vi "Nonlinear Calibration Test v2.vi"() -> ()   [LabVIEW 2009]
doc: "This example illustrates the use of a calibration grid to calibrate and correct an image for nonlinear distortion and accurate shape measurements.\n\nThis example loads the image of a calibration grid used to calibrate the system, learns the grid, then loads an image of parts acquired using the same setup. The example then corrects the image in two ways. The first method corrects the entire image and then measures the area of the coins. The second method corrects only the area of the coins and displays the difference in processing time."
uses:
  <vilib>/vision/NI_Vision_Development_Module.lvlib
panel:
  in  "Grid Descriptor":T1={"X Step"=1.0, "Y Step"=1.0, "Unit"=enum."Undefined", "Threshold Range"={"Lower value"=30.0, "Upper value"=96.0}} {"Threshold Range"."Upper value" format="%.2f"; "Threshold Range"."Lower value" format="%.2f"; "Y Step" format="%.2f"; "X Step" format="%.2f"}
  in  "Calibration Learn Setup":T3={"Distortion"=0, "Corrected Image Scaling"=0, "Corrected Image Learn ROI"=2, "Learn Error Map?"=FALSE, "Learn Correction Table?"=FALSE} {"Corrected Image Learn ROI" items=["Full Image ", "Calibration ROI", "ROI", "Calibration AND ROI", "Calibration OR ROI"]; "Corrected Image Scaling" items=["Scale to Preserve Area", "Scale to Fit"]; "Distortion" items=["Perspective", "Nonlinear"]}
  out "Bottom Image":T4(plugin-control) caption="Coins Image"
  out "Top Image":T4(plugin-control) caption="Calibration Template"
  # "1. Loads the image of a calibration grid that is used to calibrate the system."
  # "2. Learn the calibration grid. Note that this process is computation intensive and needs a fair amount of time to complete."
  # "3. Load Image of Parts acquired using the same setup."
  # "4. Correct the image and measure areas of the objects in the image."
  # "This step takes measurements in two ways.  The first calculation corrects \nthe entire image, and then takes the measurements.  The second calculation only corrects the coins, and then takes the measurements."
  # "time (ms) to correct entire image, threshold and calculate measurements"
  # "time (ms) to threshold, correct just coins, and then take measurements"
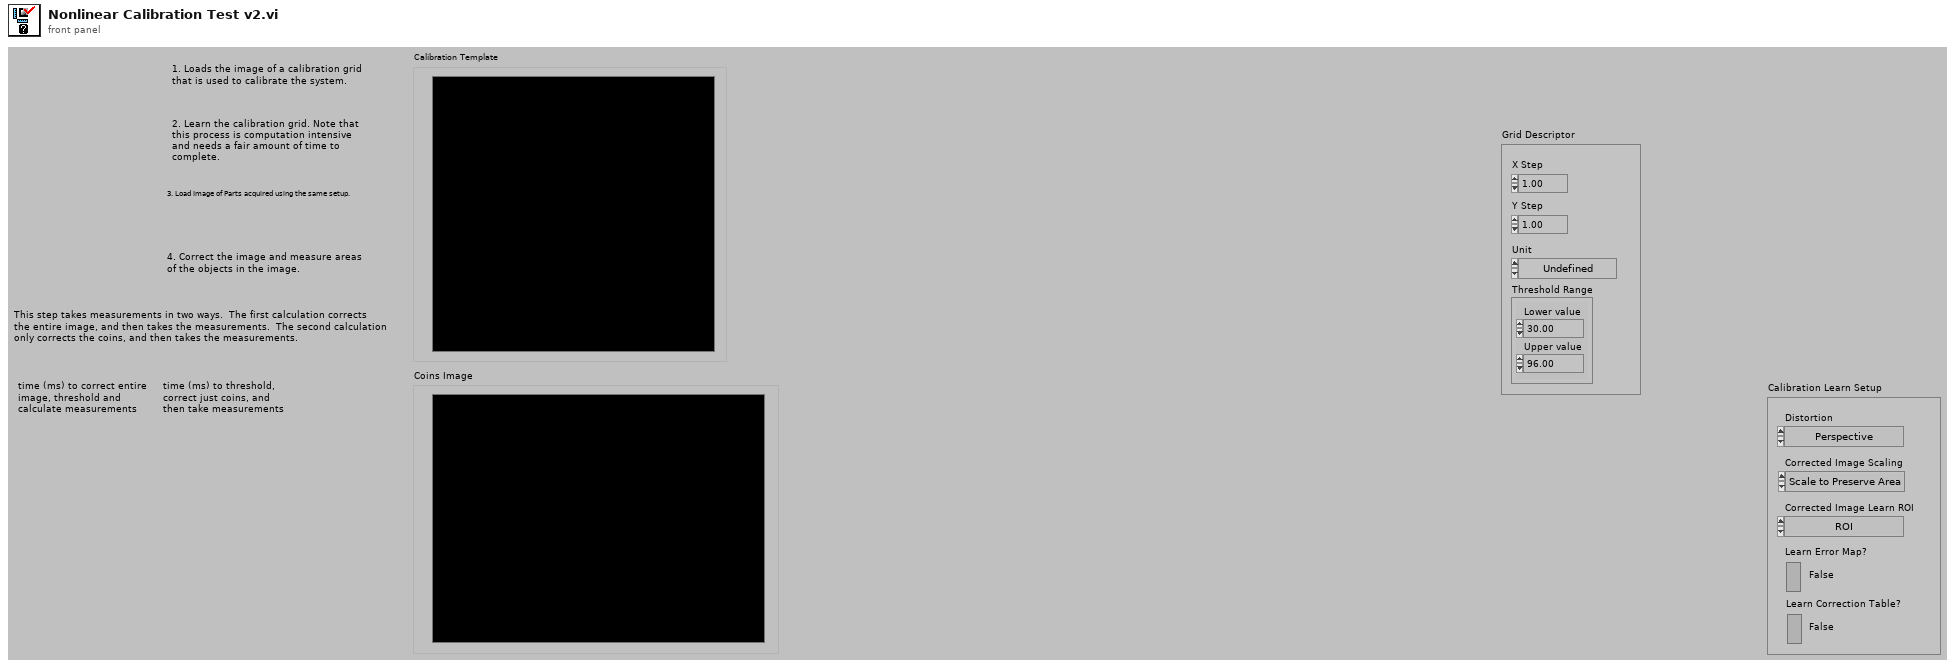
[diagram p1: front panel]
types:
  T1 = typedef "Grid Descriptor" = cluster{"X Step":sgl, "Y Step":sgl, "Unit":T2, "Threshold Range":cluster{"Lower value":sgl, "Upper value":sgl}}
  T2 = typedef "Image Unit" = enum32{"Undefined", "Angström", "Micrometer", "Millimeter", "Centimeter", "Meter", "Kilometer", "Microinch", "Inch", "Feet", "Nautical miles", "Standard miles", "Steps"}
  T3 = cluster{"Distortion":u32, "Corrected Image Scaling":u32, "Corrected Image Learn ROI":u32, "Learn Error Map?":bool, "Learn Correction Table?":bool}
  T4 = typedef "IMAQ Image.ctl" = refnum<image>
  T5 = cluster{"X Step":sgl, "Y Step":sgl, "Unit":u32, "Threshold Range":cluster{"Lower value":sgl, "Upper value":sgl}}
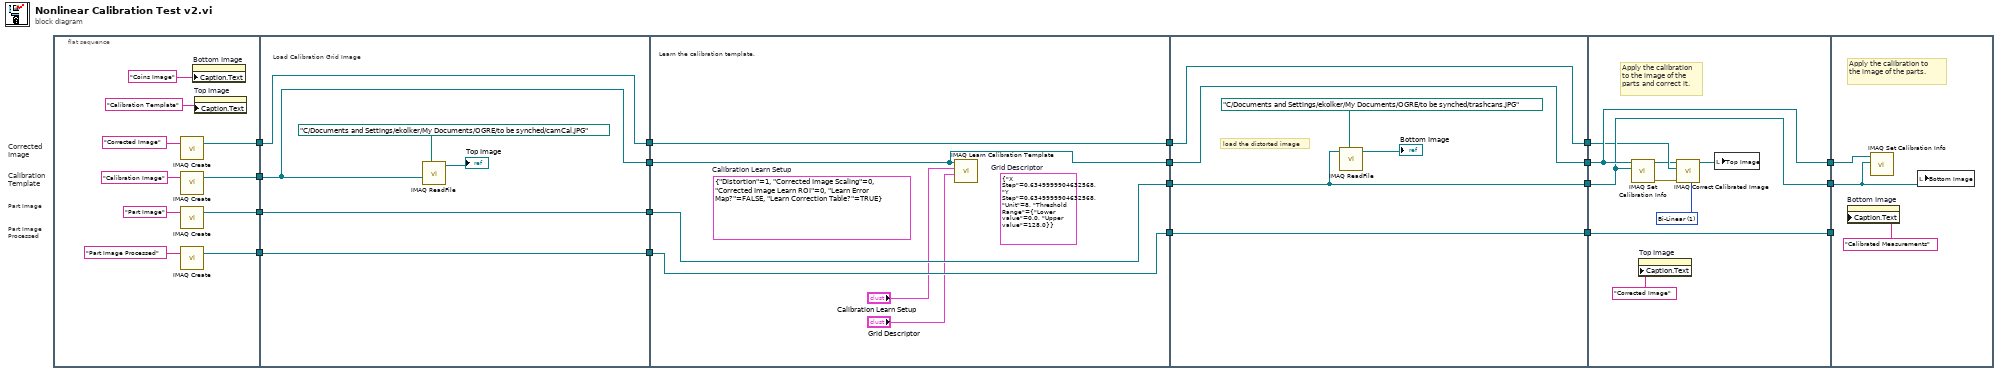
[diagram p0: block diagram]
diagram:
  # "Corrected\nImage"
  # "Part Image Processed"
  # "Calibration Template"
  # "Part Image"
  n1 = flat-sequence {
    tunnel: [w28] -> w19
    tunnel: [w26] -> w18
    tunnel: [w24] -> w17
    tunnel: [w22] -> w16
    tunnel: w19 -> [w35]
    tunnel: [w35] -> w12
    tunnel: w18 -> [w32]
    tunnel: [w32] -> w11
    tunnel: w17 -> [w34]
    tunnel: [w34] -> w10
    tunnel: w16 -> [w33]
    tunnel: [w33] -> w9
    tunnel: w12 -> [w40]
    tunnel: [w40] -> w8
    tunnel: w11 -> [w41]
    tunnel: [w41] -> w7
    tunnel: w10 -> [w39]
    tunnel: [w39] -> w6
    tunnel: w9 -> [w38]
    tunnel: [w38] -> w5
    tunnel: w8 -> [w47]
    tunnel: [w47] -> w4
    tunnel: w7 -> [w45]
    tunnel: [w45] -> w3
    tunnel: w6 -> [w44]
    tunnel: [w44] -> w2
    tunnel: w5 -> [w43]
    tunnel: [w43] -> w1
    tunnel: w4 -> [w55]
    tunnel: [w55] -> w15
    tunnel: w3 -> [w56]
    tunnel: [w56] -> w14
    tunnel: w2 -> [w54]
    tunnel: [w54] -> w13
    tunnel: w1 -> [w53]
    tunnel: w15 -> [w57]
    tunnel: w14 -> [w59]
    tunnel: w13 -> [_]
    frame #0 {
      # "Create the required images"
      n2 = call "IMAQ Create"("Image Name"="Corrected Image") -> ("New Image"=w22:T4)  [unwired: 3 in, 2 out]
      n3 = call "IMAQ Create"("Image Name"="Calibration Image") -> ("New Image"=w26:T4)  [unwired: 3 in, 2 out]
      n4 = call "IMAQ Create"("Image Name"="Part Image") -> ("New Image"=w28:T4)  [unwired: 3 in, 2 out]
      n5 = call "IMAQ Create"("Image Name"="Part Image Processed") -> ("New Image"=w24:T4)  [unwired: 3 in, 2 out]
      n6 = property on="Bottom Image" class="ImageControl"("Caption.Text"="Coins Image" ("Title")) -> ()  [unwired: 2 in, 2 out]
      n7 = property on="Top Image" class="ImageControl"("Caption.Text"="Calibration Template" ("Title")) -> ()  [unwired: 2 in, 2 out]
    }
    frame #1 {
      # "Load Calibration Grid Image"
      n8 = call "IMAQ ReadFile"("File Path"=path "C:/Documents and Settings/ekolker/My Documents/OGRE/to be synched/camCal.JPG", "Image"=w32) -> ("Image Out"=→"Top Image":T4)  [unwired: 3 in, 6 out]
    }
    frame #2 {
      (unwired) T5 {"X Step"=0.635, "Y Step"=0.635, "Unit"=8, "Threshold Range"={"Lower value"=0.0, "Upper value"=128.0}}  # Grid Descriptor
      (unwired) T3 {"Distortion"=1, "Corrected Image Scaling"=0, "Corrected Image Learn ROI"=0, "Learn Error Map?"=FALSE, "Learn Correction Table?"=TRUE}  # Calibration Learn Setup
      # "Learn the calibration template."
      n9 = call "IMAQ Learn Calibration Template"("Grid Descriptor"="Grid Descriptor", "Calibration Learn Setup"="Calibration Learn Setup", "Image"=w41) -> ()  [unwired: 4 in, 5 out]
    }
    frame #3 {
      # "load the distorted image"
      n10 = call "IMAQ ReadFile"("File Path"=path "C:/Documents and Settings/ekolker/My Documents/OGRE/to be synched/trashcans.JPG", "Image"=w47) -> ("Image Out"=→"Bottom Image":T4)  [unwired: 3 in, 6 out]
    }
    frame #4 {
      w52 = u32 1 items=["Zero Order", "Bi-Linear", "Quadratic", "Cubic Spline"] ("Interpolation Type")
      # "Apply the calibration to the image of the parts and correct it."
      n11 = call "IMAQ Set Calibration Info"("Image Dst"=w55, "Image Src"=w56) -> ("error out"=w49:errorcluster, "Calibrated Image"=w50:T4)  [unwired: 2 in, 6 out]
      n12 = property on="Top Image" class="ImageControl"("Caption.Text"="Corrected Image" ("Title")) -> ()  [unwired: 2 in, 2 out]
      n13 = call "IMAQ Correct Calibrated Image"("Interpolation Type"=w52, "error in (no error)"=w49, "Image Dst"=w53, "Image Src"=w50) -> ("Corrected Image"=w48:T4)  [unwired: 3 in, 4 out]
      n14 = local write "Top Image"(w48) -> ()
    }
    frame #5 {
      # "Apply the calibration to the image of the parts."
      n15 = property on="Bottom Image" class="ImageControl"("Caption.Text"="Calibrated Measurements" ("Title")) -> ()  [unwired: 2 in, 2 out]
      n16 = call "IMAQ Set Calibration Info"("Image Dst"=w57, "Image Src"=w59) -> ()  [unwired: 2 in, 8 out]
      n17 = local write "Bottom Image"(w57) -> ()
    }
  }
